vi "INI-FGV.vi"(4 "Raw String? (F)":bool, 5 "Write If not found?":bool, 6 "Enum":T1, 7 "Prefered Section":string, 8 "error IN":errorcluster, 9 "Path":path, 10 ">> Default Value >>":string, 11 ">> Variable Name >>":string) -> (0 "error out":errorcluster, 1 "INIConfig":refnum<class "LabVIEW-Config.lvclass">, 2 "Key?":bool, 3 "Array":string[](array[string]))   [LabVIEW 2017, in "INI-Static-Variable-Support.lvlib"]
uses:
  INI-Static-Variable-Support.lvlib
  global-csm-ini-db-change-flag.vi
  <userlib>/_NEVSTOP/Communicable State Machine(CSM)/Communicable State Machine.lvlib
  CSMSVMgr/CSM-Static-Variable-Manager.lvclass
  _Def-Ini-Variable.ctl
  _fgv-oper.ctl
  LabVIEW-Config/LabVIEW-Config.lvclass
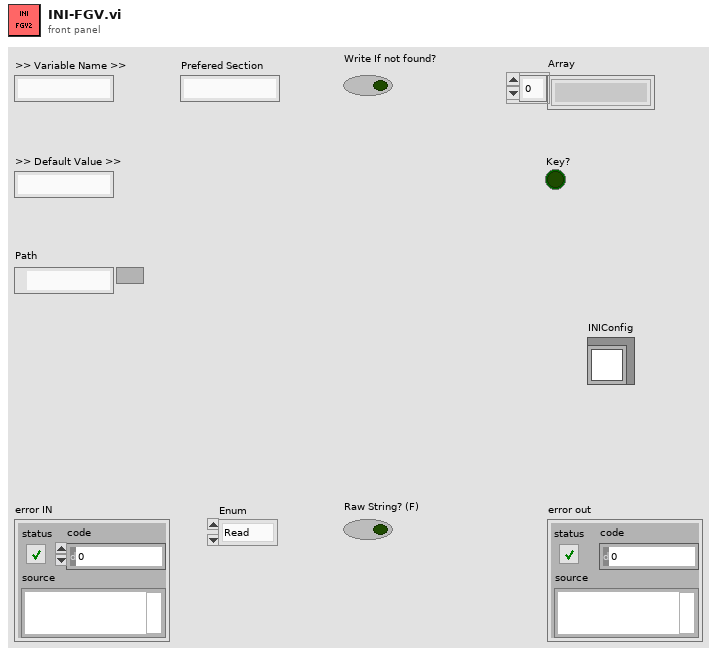
[diagram p1: front panel]
types:
  T1 = typedef "INI-Static-Variable-Support.lvlib/_fgv-oper.ctl" = enum16{"Read", "Write", "Sync", "Sessions", "List Keys", "Load", "List Files", "List Variables", "List Permanent Variables", "Mark Temp Variable as Permenent", "unload", "INIConfig(Memory)", "Reset", "Restore Variable Value"}
  T2 = typedef "INI-Static-Variable-Support.lvlib/_Def-Ini-Variable.ctl" = cluster{"Variable Name":string, "Preferred Section":string}
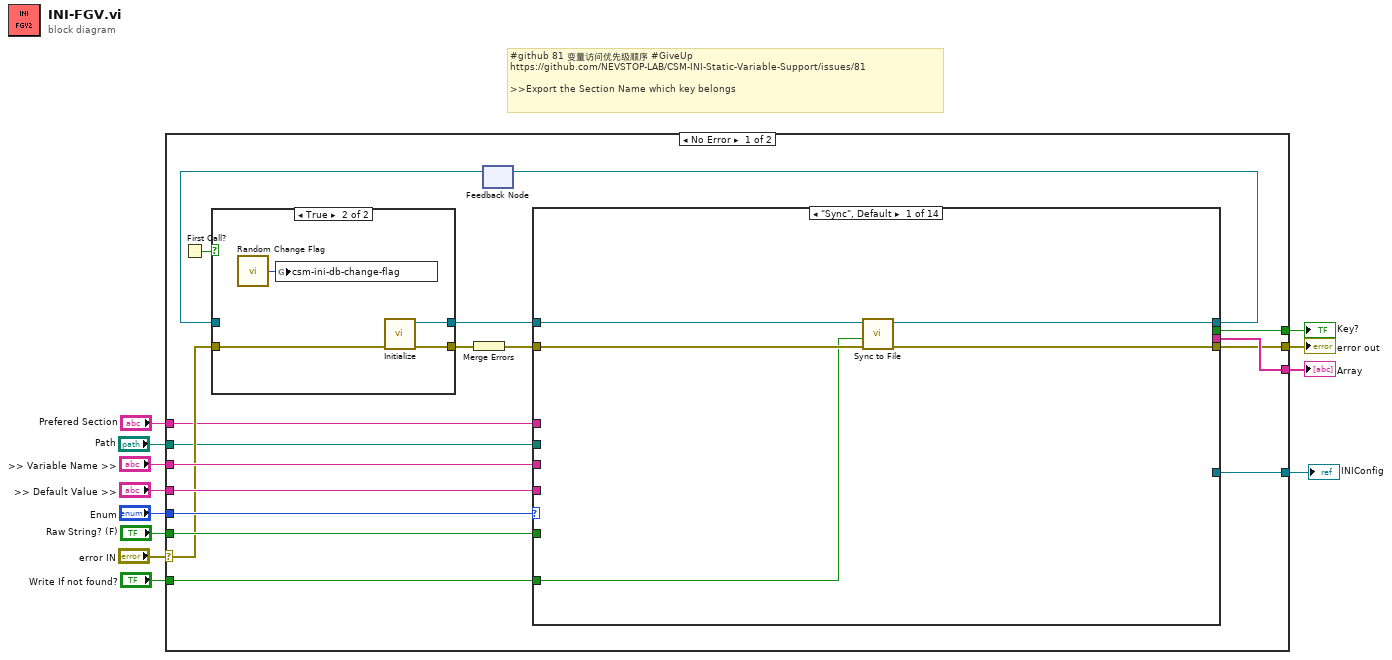
[diagram p0: block diagram]
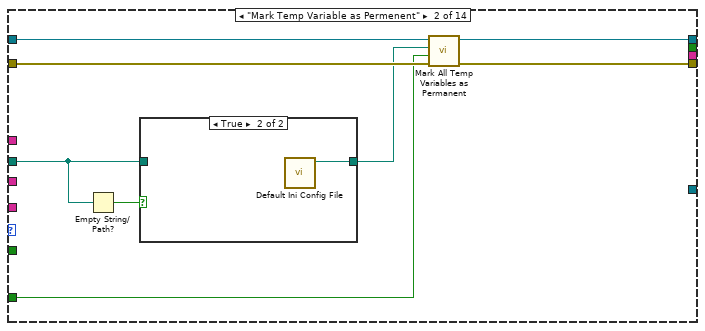
[diagram p2: hidden frame]
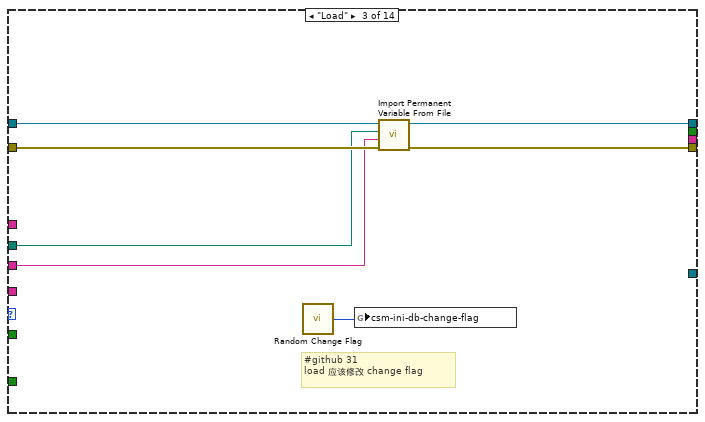
[diagram p4: hidden frame]
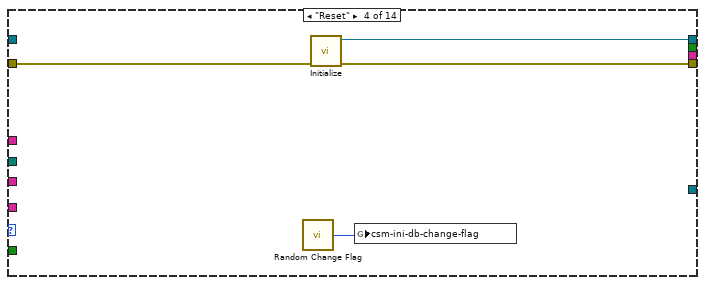
[diagram p5: hidden frame]
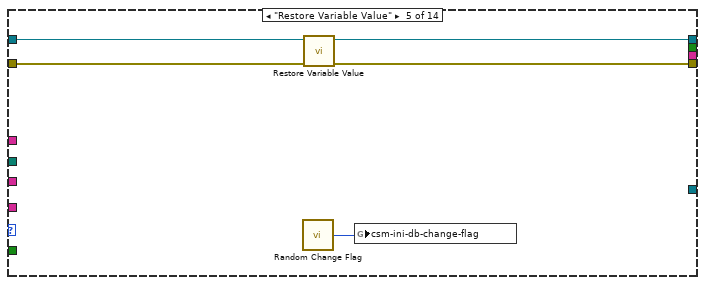
[diagram p6: hidden frame]
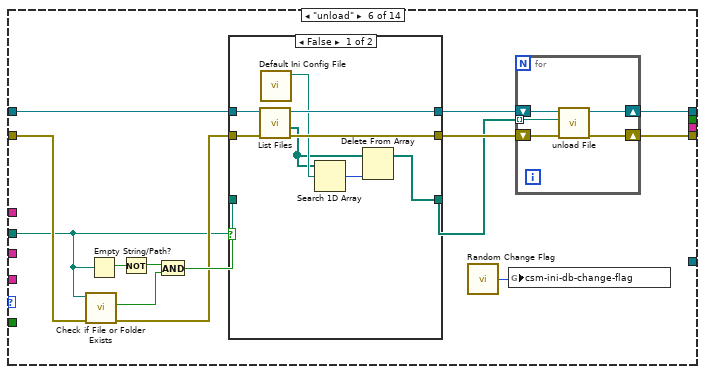
[diagram p7: hidden frame]
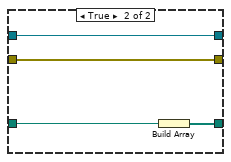
[diagram p8: hidden frame]
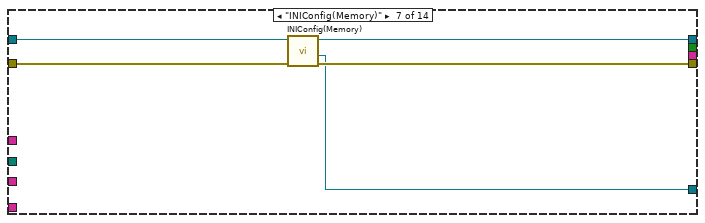
[diagram p9: hidden frame]
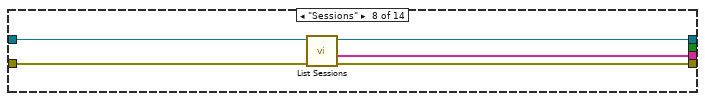
[diagram p10: hidden frame]
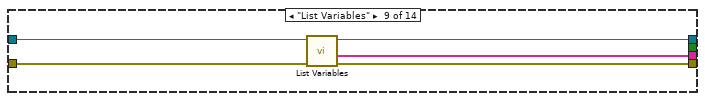
[diagram p11: hidden frame]
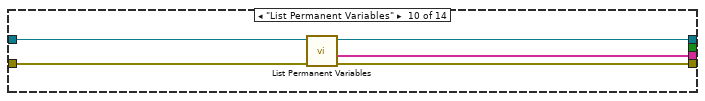
[diagram p12: hidden frame]
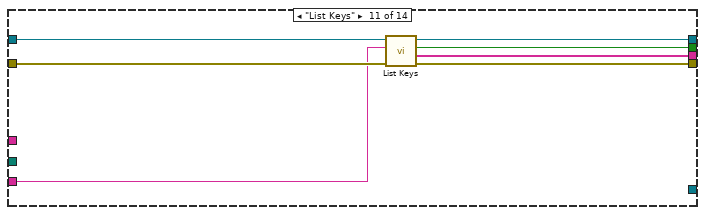
[diagram p13: hidden frame]
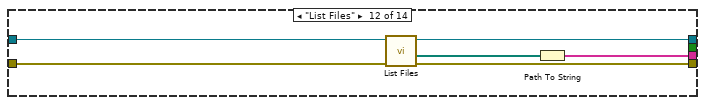
[diagram p14: hidden frame]
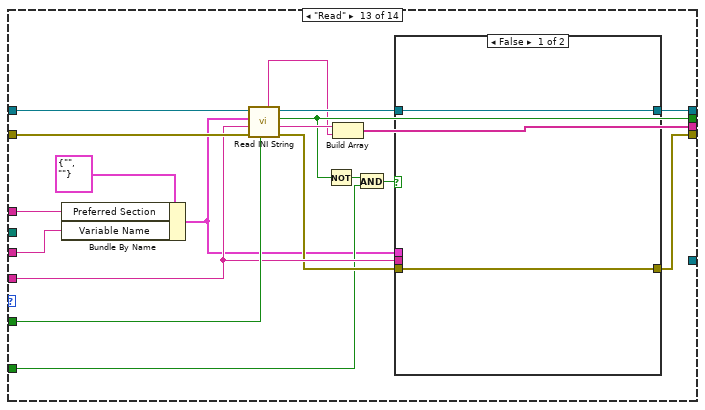
[diagram p15: hidden frame]
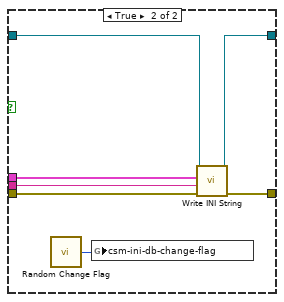
[diagram p16: hidden frame]
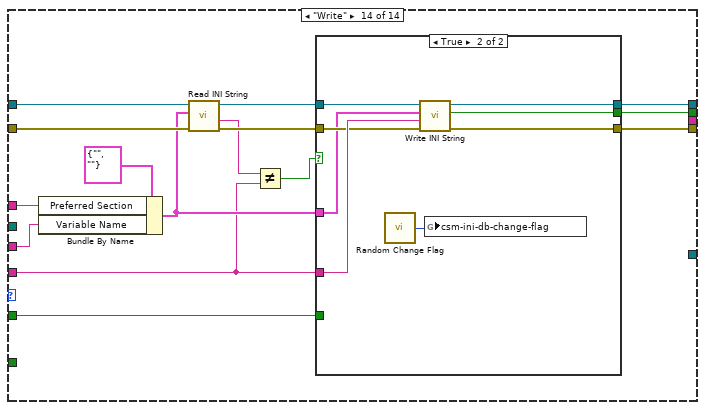
[diagram p17: hidden frame]
diagram:
  # "#github 81 变量访问优先级顺序 #GiveUp\nhttps://github.com/NEVSTOP-LAB/CSM-INI-Static-Variable-Support/issues/81\n\n>>Export the Section Name which key belongs"
  n1 = case shown="No Error" "error IN" {
    selector: "error IN" -> [w17 w185]
    tunnel: [w28 _] -> w12
    tunnel: ">> Default Value >>" -> [w27 _]
    tunnel: ">> Variable Name >>" -> [w26 _]
    tunnel: [w25 w185] -> w9
    tunnel: "Enum" -> [w20 _]
    tunnel: [w19 _] -> w7
    tunnel: "Raw String? (F)" -> [w18 _]
    tunnel: "Write If not found?" -> [w16 _]
    tunnel: "Path" -> [w15 _]
    tunnel: [w14 _] -> w2
    tunnel: "Prefered Section" -> [w13 _]
    frame No Error {
      n2 = First Call?() -> (First Call?: T/F=w24:bool)
      n3 = feedback #1() -> (w21:refnum<class "CSM-Static-Variable-Manager.lvclass">)  [unwired: 1 in]
      n4 = case shown="True" w24 {
        tunnel: [w180 w183] -> w29
        tunnel: [w179 w181] -> w23
        tunnel: w21 -> [w180 _]
        tunnel: w17 -> [w179 w182]
        frame False {
        }
        frame True {
          n5 = call <userlib>:"Random Change Flag.vi"() -> ("Random Change Flag"=w184:u64)  [unwired: 2 in]
          n6 = global write "global-csm-ini-db-change-flag.vi" "csm-ini-db-change-flag"(w184) -> ()
          n7 = call "Initialize.vi"("Error in"=w182) -> ("Error out"=w181:errorcluster, "INI-Static-Variable-Support.lvlib:CSM-Static-Variable-Manager.lvclass"=w183:refnum<class "CSM-Static-Variable-Manager.lvclass">)  [unwired: 9 in]
        }
      }
      n8 = Merge Errors(w23) -> (w30:errorcluster)
      n9 = case shown="\"Sync\", Default" w20 {
        tunnel: w30 -> [w32 w40 w49 w55 w59 w65 w97 w98 w103 w108 w117 w123 w144 w165]
        tunnel: w29 -> [w35 w43 w52 _ w60 w72 w95 w99 w104 w109 w115 w122 w132 w160]
        tunnel: [_ _ _ _ _ _ _ w100 w105 w110 w118 w120 w133 _] -> w28
        tunnel: w27 -> [_ _ _ _ _ _ _ _ _ _ _ _ w140 w154]
        tunnel: w26 -> [_ _ w46 _ _ _ _ _ _ _ w113 _ w129 w156]
        tunnel: [w33 w41 w50 w54 w57 w74 w96 w101 w106 w111 w119 w125 w138 w168] -> w25
        tunnel: [w34 w42 w51 w53 w58 w75 w94 w102 w107 w112 w114 w121 w131 w159] -> w22
        tunnel: [_ _ _ _ _ _ _ _ _ _ w116 _ w136 w167] -> w19
        tunnel: w18 -> [_ _ _ _ _ _ _ _ _ _ _ _ w142 w166]
        tunnel: w16 -> [w31 w36 _ _ _ _ _ _ _ _ _ _ w134 _]
        tunnel: w15 -> [_ w38 w48 _ _ w62 _ _ _ _ _ _ _ _]
        tunnel: [_ _ _ _ _ _ w93 _ _ _ _ _ _ _] -> w14
        tunnel: w13 -> [_ _ _ _ _ _ _ _ _ _ _ _ w128 w157]
        frame "Sync", Default {
          n10 = call "Sync to File.vi"("error in (no error)"=w32, "Write Reference?(F)"=w31, "CSM-Static-Variable-Manager in"=w35) -> ("error out"=w33:errorcluster, "CSM-Static-Variable-Manager out"=w34:refnum<class "CSM-Static-Variable-Manager.lvclass">)  [unwired: 7 in]
        }
        frame "Mark Temp Variable as Permenent" {
          n11 = Empty String/Path?(string/path=w38) -> (empty?=w39:bool)
          n12 = case shown="True" w39 {
            tunnel: w38 -> [w44 _]
            tunnel: [w44 w45] -> w37
            frame False {
            }
            frame True {
              n13 = call "Default Ini Config File.vi"() -> ("appended path"=w45:path)  [unwired: 11 in]
            }
          }
          n14 = call "Mark All Temp Variables as Permanent.vi"("error in (no error)"=w40, "SyncRef?(F)"=w36, "Path"=w37, "CSM-Static-Variable-Manager in"=w43) -> ("error out"=w41:errorcluster, "CSM-Static-Variable-Manager out"=w42:refnum<class "CSM-Static-Variable-Manager.lvclass">)  [unwired: 6 in]
        }
        frame "Load" {
          # "#github 31\nload 应该修改 change flag"
          n15 = call <userlib>:"Random Change Flag.vi"() -> ("Random Change Flag"=w47:u64)  [unwired: 2 in]
          n16 = global write "global-csm-ini-db-change-flag.vi" "csm-ini-db-change-flag"(w47) -> ()
          n17 = call "Import Permanent Variable From File.vi"("error in (no error)"=w49, "section postfix"=w46, "Path"=w48, "CSM-Static-Variable-Manager in"=w52) -> ("error out"=w50:errorcluster, "CSM-Static-Variable-Manager out"=w51:refnum<class "CSM-Static-Variable-Manager.lvclass">)  [unwired: 6 in]
        }
        frame "Reset" {
          n18 = call <userlib>:"Random Change Flag.vi"() -> ("Random Change Flag"=w56:u64)  [unwired: 2 in]
          n19 = call "Initialize.vi"("Error in"=w55) -> ("Error out"=w54:errorcluster, "INI-Static-Variable-Support.lvlib:CSM-Static-Variable-Manager.lvclass"=w53:refnum<class "CSM-Static-Variable-Manager.lvclass">)  [unwired: 9 in]
          n20 = global write "global-csm-ini-db-change-flag.vi" "csm-ini-db-change-flag"(w56) -> ()
        }
        frame "Restore Variable Value" {
          n21 = call <userlib>:"Random Change Flag.vi"() -> ("Random Change Flag"=w61:u64)  [unwired: 2 in]
          n22 = call "Restore Variable Value.vi"("error in (no error)"=w59, "CSM-Static-Variable-Manager in"=w60) -> ("error out"=w57:errorcluster, "CSM-Static-Variable-Manager out"=w58:refnum<class "CSM-Static-Variable-Manager.lvclass">)  [unwired: 8 in]
          n23 = global write "global-csm-ini-db-change-flag.vi" "csm-ini-db-change-flag"(w61) -> ()
        }
        frame "unload" {
          n24 = call <vilib>:"Check if File or Folder Exists.vi"("error in (no error)"=w65, "path"=w62) -> ("error out"=w64:errorcluster, "file or folder exists?"=w67:bool)  [unwired: 7 in, 1 out]
          n25 = Empty String/Path?(string/path=w62) -> (empty?=w69:bool)
          n26 = Not(x=w69) -> (.not. x?=w68:bool)
          n27 = And(x=w68, y=w67) -> (x .and. y?=w66:bool)
          n28 = case shown="False" w66 {
            tunnel: w72 -> [w83 w86]
            tunnel: [w82 w86] -> w71
            tunnel: [w81 w85] -> w70
            tunnel: w64 -> [w80 w85]
            tunnel: [w76 w84] -> w63
            tunnel: w62 -> [_ w87]
            frame False {
              n29 = call "List Files.vi"("error in (no error)"=w80, "CSM-Static-Variable-Manager in"=w83) -> ("error out"=w81:errorcluster, "File List"=w77:path[], "CSM-Static-Variable-Manager out"=w82:refnum<class "CSM-Static-Variable-Manager.lvclass">)  [unwired: 7 in]
              n30 = call "Default Ini Config File.vi"() -> ("appended path"=w79:path)  [unwired: 11 in]
              n31 = Search 1D Array(1D array=w77, element=w79) -> (index of element=w78:i32)  [unwired: 1 in]
              n32 = Delete From Array(array=w77, index=w78) -> (array with subset deleted=w76:path[])  [unwired: 1 in, 1 out]
            }
            frame True {
              n33 = Build Array(w87) -> (w84:path[])
            }
          }
          n34 = call <userlib>:"Random Change Flag.vi"() -> ("Random Change Flag"=w73:u64)  [unwired: 2 in]
          n35 = global write "global-csm-ini-db-change-flag.vi" "csm-ini-db-change-flag"(w73) -> ()
          n36 = for {
            tunnel: w63 -> [w88] mode=indexing
            shift-right: [w92] -> w75
            shift-left: w71 -> [w90]
            shift-right: [w91] -> w74
            shift-left: w70 -> [w89]
            n37 = call "unload File.vi"("error in (no error)"=w89, "Path"=w88, "CSM-Static-Variable-Manager in"=w90) -> ("error out"=w91:errorcluster, "CSM-Static-Variable-Manager out"=w92:refnum<class "CSM-Static-Variable-Manager.lvclass">)  [unwired: 7 in]
          }
        }
        frame "INIConfig(Memory)" {
          n38 = call "INIConfig(Memory).vi"("error in (no error)"=w97, "CSM-Static-Variable-Manager in"=w95) -> ("error out"=w96:errorcluster, "Memory"=w93:refnum<class "LabVIEW-Config.lvclass">, "CSM-Static-Variable-Manager out"=w94:refnum<class "CSM-Static-Variable-Manager.lvclass">)  [unwired: 7 in]
        }
        frame "Sessions" {
          n39 = call "List Sessions.vi"("error in (no error)"=w98, "CSM-Static-Variable-Manager in"=w99) -> ("error out"=w101:errorcluster, "Array"=w100:string[], "CSM-Static-Variable-Manager out"=w102:refnum<class "CSM-Static-Variable-Manager.lvclass">)  [unwired: 7 in]
        }
        frame "List Variables" {
          n40 = call "List Variables.vi"("error in (no error)"=w103, "CSM-Static-Variable-Manager in"=w104) -> ("error out"=w106:errorcluster, "Variables"=w105:string[], "CSM-Static-Variable-Manager out"=w107:refnum<class "CSM-Static-Variable-Manager.lvclass">)  [unwired: 7 in]
        }
        frame "List Permanent Variables" {
          n41 = call "List Permanent Variables.vi"("error in (no error)"=w108, "CSM-Static-Variable-Manager in"=w109) -> ("error out"=w111:errorcluster, "Permanent Variables"=w110:string[], "CSM-Static-Variable-Manager out"=w112:refnum<class "CSM-Static-Variable-Manager.lvclass">)  [unwired: 7 in]
        }
        frame "List Keys" {
          n42 = call "List Keys.vi"("error in (no error)"=w117, "Section Name"=w113, "CSM-Static-Variable-Manager in"=w115) -> ("error out"=w119:errorcluster, "Array"=w118:string[], "Key?"=w116:bool, "CSM-Static-Variable-Manager out"=w114:refnum<class "CSM-Static-Variable-Manager.lvclass">)  [unwired: 5 in]
        }
        frame "List Files" {
          n43 = call "List Files.vi"("error in (no error)"=w123, "CSM-Static-Variable-Manager in"=w122) -> ("error out"=w125:errorcluster, "File List"=w124:path[], "CSM-Static-Variable-Manager out"=w121:refnum<class "CSM-Static-Variable-Manager.lvclass">)  [unwired: 7 in]
          n44 = Path To String(path=w124) -> (string=w120:string[])
        }
        frame "Read" {
          n45 = Bundle By Name(cluster=T2 {"Variable Name"="", "Preferred Section"=""} ("Variable"), "Preferred Section"=w128, "Variable Name"=w129) -> (w127:T2)
          n46 = call "Read INI String.vi"("Force Default Session?(F)"=w142, "error in (no error)"=w144, "Default"=w140, "Variable"=w127, "CSM-Static-Variable-Manager in"=w132) -> ("error out"=w139:errorcluster, "Content"=w143:string, "Key Found?"=w136:bool, "CSM-Static-Variable-Manager out"=w141:refnum<class "CSM-Static-Variable-Manager.lvclass">, "Section Name"=w126:string)  [unwired: 2 in]
          n47 = Not(x=w136) -> (.not. x?=w135:bool)
          n48 = Build Array(w143, w126) -> (w133:string[])
          n49 = And(x=w135, y=w134) -> (x .and. y?=w137:bool)
          n50 = case shown="False" w137 {
            tunnel: w141 -> [w146 w147]
            tunnel: [w146 w153] -> w131
            tunnel: w127 -> [_ w152]
            tunnel: w140 -> [_ w151]
            tunnel: w139 -> [w145 w150]
            tunnel: [w145 w149] -> w138
            frame False {
            }
            frame True {
              n51 = call <userlib>:"Random Change Flag.vi"() -> ("Random Change Flag"=w148:u64)  [unwired: 2 in]
              n52 = global write "global-csm-ini-db-change-flag.vi" "csm-ini-db-change-flag"(w148) -> ()
              n53 = call "Write INI String.vi"("error in (no error)"=w150, "Content"=w151, "Variable"=w152, "CSM-Static-Variable-Manager in"=w147) -> ("error out"=w149:errorcluster, "CSM-Static-Variable-Manager out"=w153:refnum<class "CSM-Static-Variable-Manager.lvclass">)  [unwired: 5 in, 1 out]
            }
          }
        }
        frame "Write" {
          n54 = Bundle By Name(cluster=T2 {"Variable Name"="", "Preferred Section"=""} ("Variable"), "Preferred Section"=w157, "Variable Name"=w156) -> (w155:T2)
          n55 = call "Read INI String.vi"("error in (no error)"=w165, "Variable"=w155, "CSM-Static-Variable-Manager in"=w160) -> ("error out"=w163:errorcluster, "Content"=w162:string, "CSM-Static-Variable-Manager out"=w164:refnum<class "CSM-Static-Variable-Manager.lvclass">)  [unwired: 4 in, 2 out]
          n56 = Not Equal?(x=w162, y=w154) -> (x != y?=w161:bool)
          n57 = case shown="True" w161 {
            tunnel: [w170 w178] -> w168
            tunnel: [w169 w177] -> w159
            tunnel: w154 -> [_ w176]
            tunnel: [_ w175] -> w167
            tunnel: w166 -> [_ _]
            tunnel: w164 -> [w169 w171]
            tunnel: w163 -> [w170 w174]
            tunnel: w155 -> [_ w173]
            frame False {
            }
            frame True {
              n58 = call <userlib>:"Random Change Flag.vi"() -> ("Random Change Flag"=w172:u64)  [unwired: 2 in]
              n59 = call "Write INI String.vi"("error in (no error)"=w174, "Content"=w176, "Variable"=w173, "CSM-Static-Variable-Manager in"=w171) -> ("error out"=w178:errorcluster, "Key Replaced?"=w175:bool, "CSM-Static-Variable-Manager out"=w177:refnum<class "CSM-Static-Variable-Manager.lvclass">)  [unwired: 5 in]
              n60 = global write "global-csm-ini-db-change-flag.vi" "csm-ini-db-change-flag"(w172) -> ()
            }
          }
        }
      }
      n61 = feedback-in #1(w22) -> ()
    }
    frame Error {
    }
  }
  "Array" <- w12
  "error out" <- w9
  "Key?" <- w7
  "INIConfig" <- w2
